vi "parse.series.header.vi"(7 "series body":string, 8 "error in (no error)":errorcluster, 11 "ComicVine_class in":refnum<class "series_class.lvclass">) -> (0 "error out":errorcluster, 3 "ComicVine_class out":refnum<class "series_class.lvclass">)   [LabVIEW 2024, in "series_class.lvclass"]
uses:
  series_class.lvclass
  series_class.lvclass/series_class.ctl
  <vilib>/Utility/error.llb/Trim Whitespace.vi
  <vilib>/Utility/error.llb/Trim Whitespace One-Sided.vi
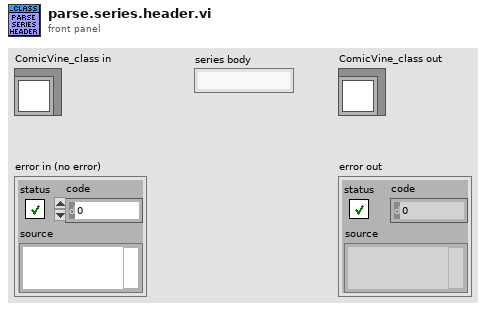
[diagram p1: front panel]
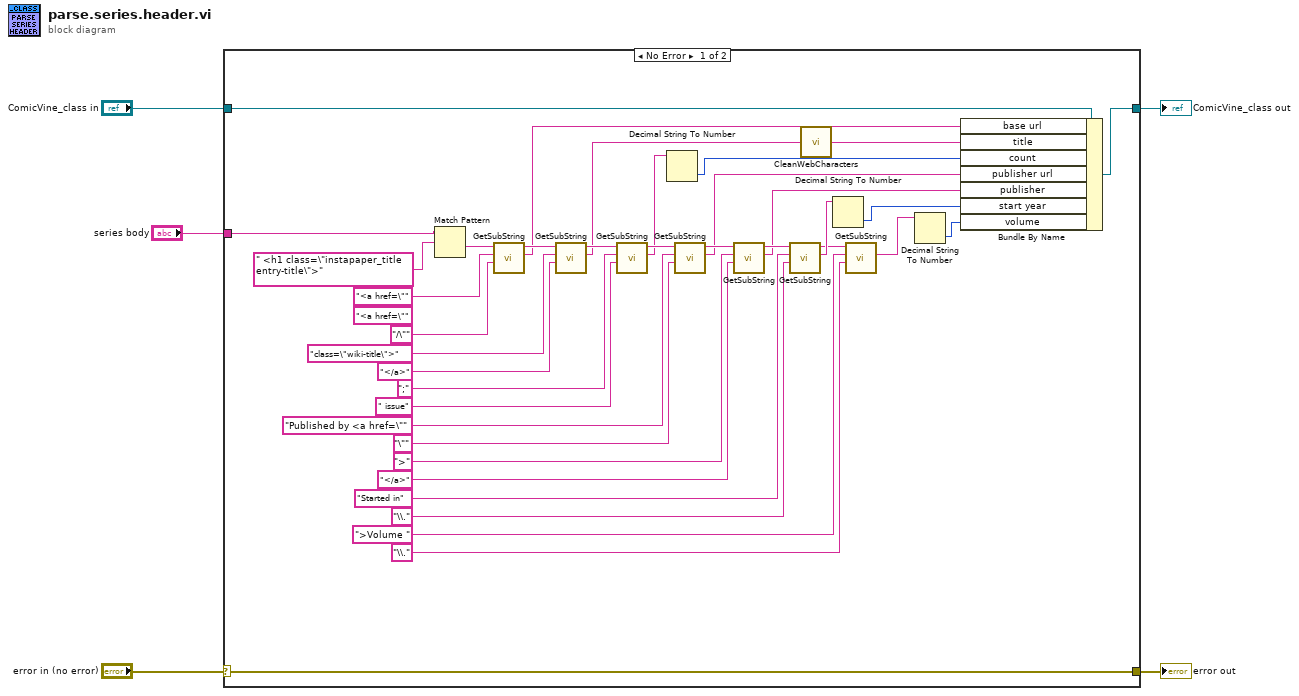
[diagram p0: block diagram]
diagram:
  n1 = case shown="No Error" "error in (no error)" {
    selector: "error in (no error)" -> [w42 w44]
    tunnel: [w42 w44] -> w4
    tunnel: [w15 w43] -> w2
    tunnel: "ComicVine_class in" -> [w16 w43]
    tunnel: "series body" -> [w6 _]
    frame No Error {
      (unwired) "<a href=\"" ("Start Search")
      n2 = Match Pattern(string=w6, regular expression=" <h1 class=\"instapaper_title entry-title\">") -> (after substring=w39:string)  [unwired: 1 in, 3 out]
      n3 = call "GetSubString.vi"("End Search"="/\"" ("Start Search"), "Start Search"="<a href=\"", "String In"=w39) -> ("Match"=w14:string, "Following String Out"=w37:string)  [unwired: 6 in, 1 out]
      n4 = call "GetSubString.vi"("End Search"="</a>" ("Start Search"), "Start Search"="class=\"wiki-title\">", "String In"=w37) -> ("Match"=w13:string, "Following String Out"=w34:string)  [unwired: 6 in, 1 out]
      n5 = call "GetSubString.vi"("End Search"=" issue" ("Start Search"), "Start Search"=";", "String In"=w34) -> ("Match"=w17:string, "Following String Out"=w31:string)  [unwired: 6 in, 1 out]
      n6 = Decimal String To Number(string=w17) -> (number=w12:i32)  [unwired: 2 in, 1 out]
      n7 = call "GetSubString.vi"("End Search"="\"" ("Start Search"), "Start Search"="Published by <a href=\"", "String In"=w31) -> ("Match"=w11:string, "Following String Out"=w28:string)  [unwired: 6 in, 1 out]
      n8 = call "GetSubString.vi"("End Search"="</a>" ("Start Search"), "Start Search"=">", "String In"=w28) -> ("Match"=w10:string, "Following String Out"=w25:string)  [unwired: 6 in, 1 out]
      n9 = call "GetSubString.vi"("End Search"="\\." ("Start Search"), "Start Search"="Started in", "String In"=w25) -> ("Match"=w22:string, "Following String Out"=w21:string)  [unwired: 6 in, 1 out]
      n10 = call "CleanWebCharacters.vi"("string in"=w13) -> ("string out"=w7:string)
      n11 = Decimal String To Number(string=w22) -> (number=w9:i32)  [unwired: 2 in, 1 out]
      n12 = call "GetSubString.vi"("End Search"="\\." ("Start Search"), "Start Search"=">Volume ", "String In"=w21) -> ("Match"=w18:string)  [unwired: 6 in, 2 out]
      n13 = Decimal String To Number(string=w18) -> (number=w8:i32)  [unwired: 2 in, 1 out]
      n14 = Bundle By Name(cluster=w16, "base url"=w14, "title"=w7, "count"=w12, "publisher url"=w11, "publisher"=w10, "start year"=w9, "volume"=w8) -> (w15:refnum<class "series_class.lvclass">)
    }
    frame Error {
    }
  }
  "error out" <- w4
  "ComicVine_class out" <- w2
